vi "IMAQdx-Names.vi"(8 "error in (no error)":errorcluster, 11 "exactCameraName":string="Point Gray Camera") -> (0 "error out":errorcluster, 2 "Defaults":string, 3 "shortcuts":cluster{"ExposureTime":string, "Gain":string})   [LabVIEW 2011]
panel:
  # "pointgray,basler,  martixvision,"
  # "! keine leerzeichen!"
  # "exposure"
  # "autoexposure"
  # "gain"
  # "autogain?"
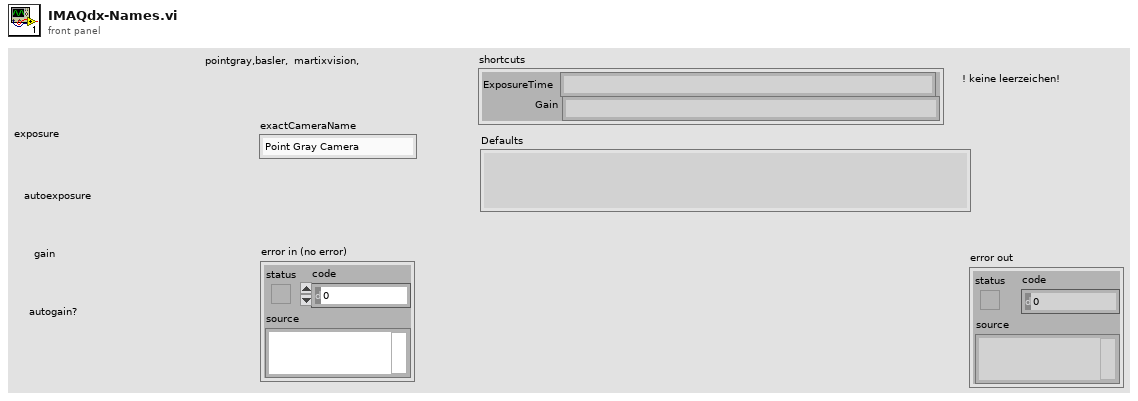
[diagram p1: front panel]
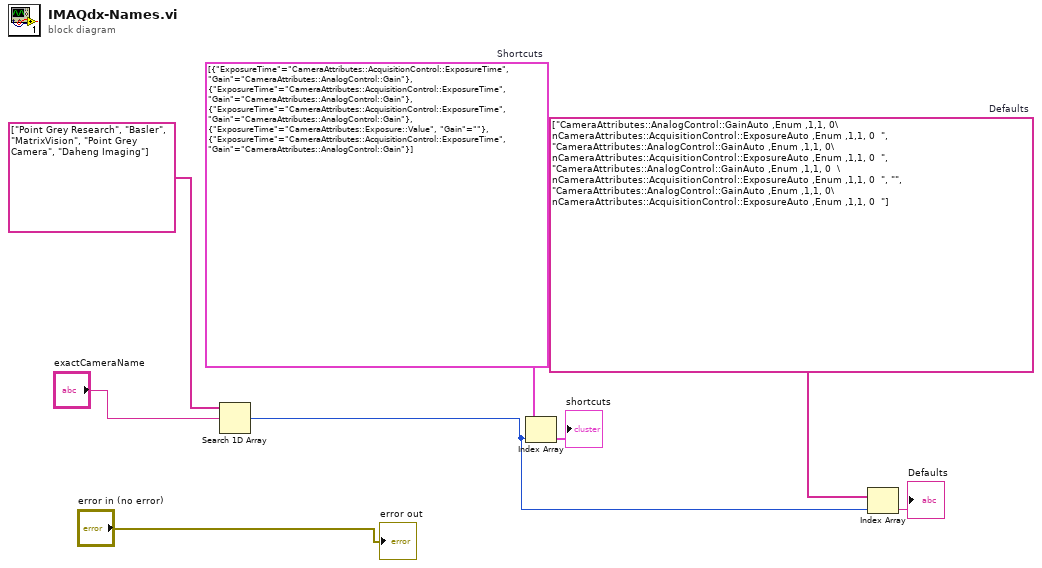
[diagram p0: block diagram]
diagram:
  w6 = cluster{"ExposureTime":string, "Gain":string}[] [{"ExposureTime"="CameraAttributes::AcquisitionControl::ExposureTime", "Gain"="CameraAttributes::AnalogControl::Gain"}, {"ExposureTime"="CameraAttributes::AcquisitionControl::ExposureTime", "Gain"="CameraAttributes::AnalogControl::Gain"}, {"ExposureTime"="CameraAttributes::AcquisitionControl::ExposureTime", "Gain"="CameraAttributes::AnalogControl::Gain"}, {"ExposureTime"="CameraAttributes::Exposure::Value", "Gain"=""}, {"ExposureTime"="CameraAttributes::AcquisitionControl::ExposureTime", "Gain"="CameraAttributes::AnalogControl::Gain"}]  # Shortcuts
  w4 = string[] ["CameraAttributes::AnalogControl::GainAuto ,Enum ,1,1, 0\nCameraAttributes::AcquisitionControl::ExposureAuto ,Enum ,1,1, 0  ", "CameraAttributes::AnalogControl::GainAuto ,Enum ,1,1, 0\nCameraAttributes::AcquisitionControl::ExposureAuto ,Enum ,1,1, 0  ", "CameraAttributes::AnalogControl::GainAuto ,Enum ,1,1, 0  \nCameraAttributes::AcquisitionControl::ExposureAuto ,Enum ,1,1, 0  ", "", "CameraAttributes::AnalogControl::GainAuto ,Enum ,1,1, 0\nCameraAttributes::AcquisitionControl::ExposureAuto ,Enum ,1,1, 0  "]  # Defaults
  n1 = Search 1D Array(1D array=string[] ["Point Grey Research", "Basler", "MatrixVision", "Point Grey Camera", "Daheng Imaging"] ("VendorName"), element="exactCameraName") -> (index of element=w3:i32)  [unwired: 1 in]
  n2 = Index Array(array=w6, index=w3) -> (element=→"shortcuts":cluster{"ExposureTime":string, "Gain":string})
  n3 = Index Array(array=w4, index=w3) -> (element=→"Defaults":string)
  "error out" <- "error in (no error)"
